vi "Write Messenger Reference.vi"(8 "error in (no error)":errorcluster, 10 "Messenger Reference":refnum<data-value>, 11 "Composite Task in":refnum<class "Linked List Task.lvclass">) -> (0 "error out":errorcluster, 3 "Composite Task out":refnum<class "Linked List Task.lvclass">)   [LabVIEW 2024, in "Linked List Task.lvclass"]
uses:
  Linked List Task.lvclass
  Linked List Task.lvclass/Linked List Task.ctl
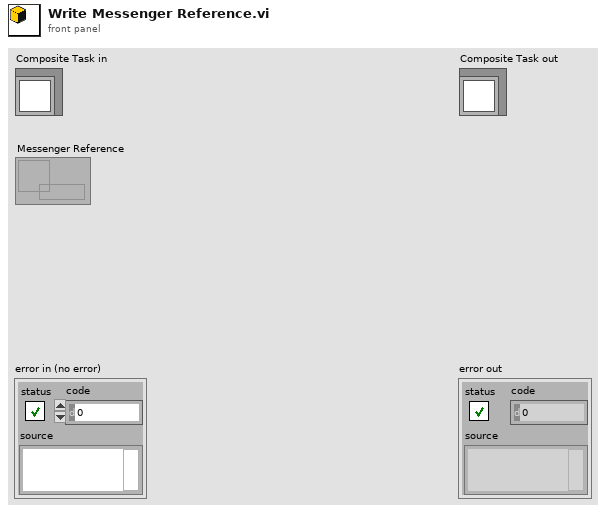
[diagram p1: front panel]
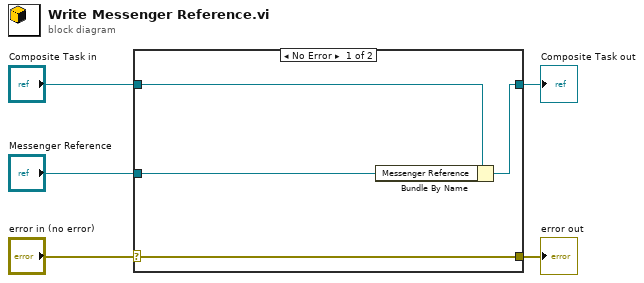
[diagram p0: block diagram]
diagram:
  n1 = case shown="No Error" "error in (no error)" {
    selector: "error in (no error)" -> [w9 w10]
    tunnel: [w9 w10] -> w4
    tunnel: [w7 w11] -> w2
    tunnel: "Composite Task in" -> [w8 w11]
    tunnel: "Messenger Reference" -> [w6 _]
    frame No Error {
      n2 = Bundle By Name(cluster=w8, "Messenger Reference"=w6) -> (w7:refnum<class "Linked List Task.lvclass">)
    }
    frame Error {
    }
  }
  "error out" <- w4
  "Composite Task out" <- w2
